vi "List Channels.vi"(8 "error in (no error)":errorcluster, 11 "E2E editor node in":refnum<data-value>) -> (0 "error out":errorcluster, 1 "Output Channels":refnum<class "TBM channel.lvclass">[](array[class]), 2 "Input Channels":refnum<class "TBM channel.lvclass">[](array[class]), 3 "E2E editor node out":refnum<data-value>)   [LabVIEW 2015, in "E2E Tag Exchange editor node.lvclass"]
uses:
  E2E Tag Exchange editor node.lvclass
  <vilib>/NI/Tag Bus Module Framework/channel/TBM channel.lvclass
  <vilib>/NI/Tag Bus Module Framework/channel/channel classification.ctl
  E2E Tag Exchange editor node.lvclass/E2E Tag Exchange editor node.ctl
  module/configuration/E2E Tag Exchange configuration.lvclass
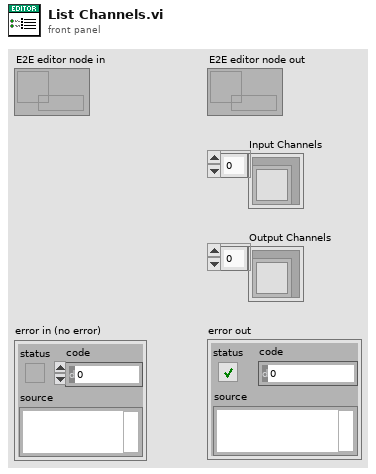
[diagram p1: front panel]
types:
  T1 = typedef "TBM channel.lvclass/channel classification.ctl" = enum16{"input data", "output data", "processing parameter", "processing result"}
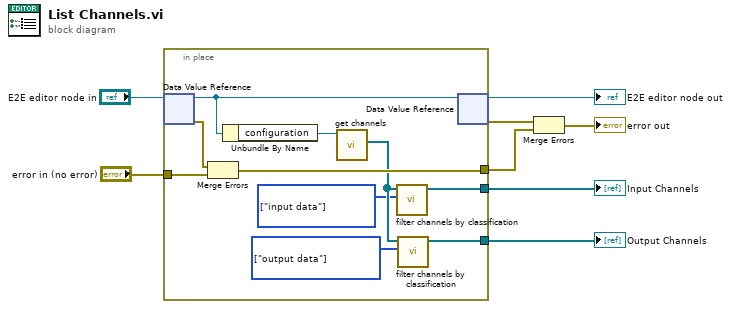
[diagram p0: block diagram]
diagram:
  n1 = in-place {
    in-place-border: "error in (no error)" -> [w16]
    in-place-border: [w14] -> w5
    in-place-border: [w10] -> w2
    in-place-border: [w9] -> w1
    w11 = T1[] [enum."output data"] items=["input data", "output data", "processing parameter", "processing result"] ("allowed classifications")
    w12 = T1[] [enum."input data"] items=["input data", "output data", "processing parameter", "processing result"] ("allowed classifications")
    n2 = in-place-dvr #1("E2E editor node in") -> (w18:refnum<class "E2E Tag Exchange editor node.lvclass">, w17:errorcluster)
    n3 = Merge Errors(w17, w16) -> (w14:errorcluster)
    n4 = Unbundle By Name(w18) -> ("configuration"=w15:refnum<class "E2E Tag Exchange configuration.lvclass">)
    n5 = call-dynamic "get channels.vi"("E2E configuration in"=w15) -> ("channels"=w13:refnum<class "TBM channel.lvclass">[])  [unwired: 9 in, 1 out]
    n6 = call <vilib>:"filter channels by classification.vi"("allowed classifications"=w12, "channels in"=w13) -> ("channels out"=w10:refnum<class "TBM channel.lvclass">[])  [unwired: 9 in]
    n7 = call <vilib>:"filter channels by classification.vi"("allowed classifications"=w11, "channels in"=w13) -> ("channels out"=w9:refnum<class "TBM channel.lvclass">[])  [unwired: 9 in]
    n8 = in-place-dvr #1(w18) -> (→"E2E editor node out":refnum<data-value>, w6:errorcluster)
  }
  "Input Channels" <- w2
  "Output Channels" <- w1
  n9 = Merge Errors(w6, w5) -> (→"error out":errorcluster)
